vi "extract_exe.vi"(4 "files_to_extract (relative) []":path[](array[path]), 6 "quiet?":bool=TRUE, 8 "error in (no error)":errorcluster, 9 "preview?":bool, 10 "target_path in":path, 11 "archive_path (file_dialog)":path) -> (0 "error out":errorcluster, 1 "files []":path[](array[path]), 2 "target_path out":path, 3 "archive_path out":path)   [LabVIEW 2015, in "lv-bin-7zip.lvlib"]
uses:
  lv-bin-7zip.lvlib
  <userlib>/antonio-alexander/lv-bin/public/api/v1/v1.lvlib
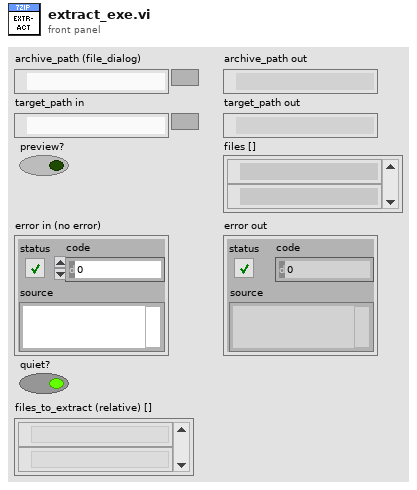
[diagram p1: front panel]
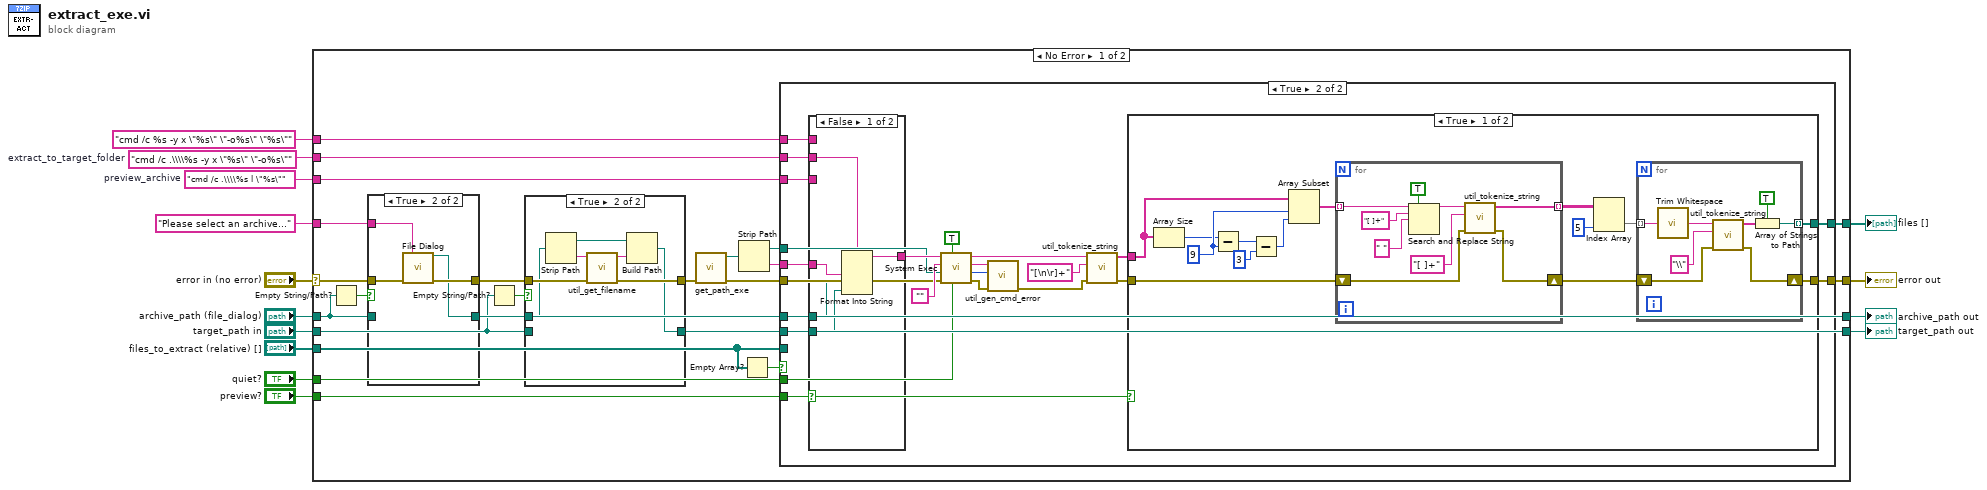
[diagram p0: block diagram]
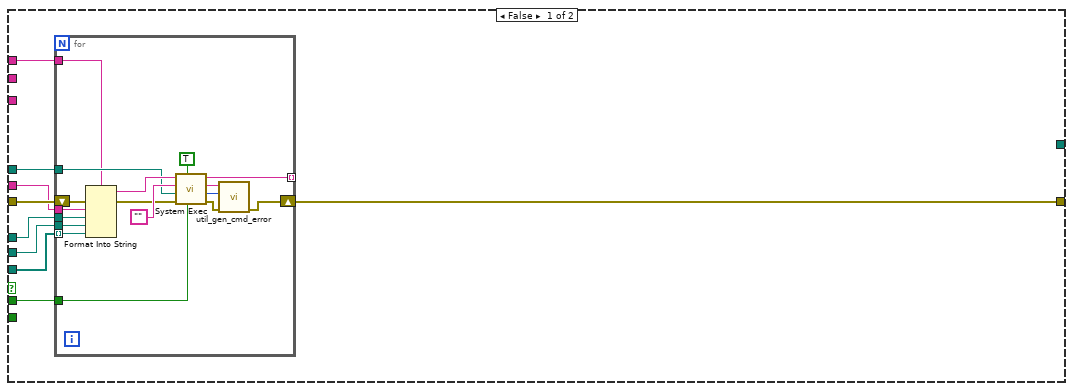
[diagram p4: hidden frame]
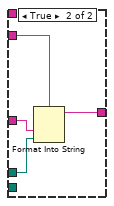
[diagram p5: hidden frame]
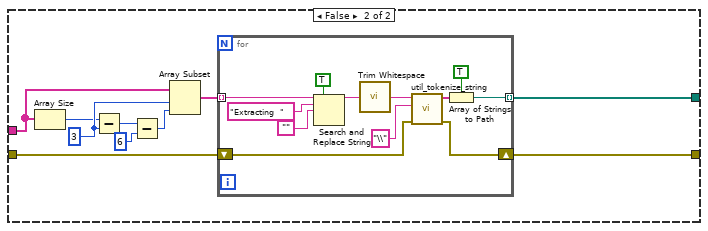
[diagram p6: hidden frame]
diagram:
  w5 = "cmd /c .\\\\%s l \"%s\""  # preview_archive
  w6 = "cmd /c .\\\\%s -y x \"%s\" \"-o%s\""  # extract_to_target_folder
  n1 = case shown="No Error" "error in (no error)" {
    selector: "error in (no error)" -> [w34 w163]
    tunnel: [w22 w163] -> w13
    tunnel: "target_path in" -> [w20 _]
    tunnel: "archive_path (file_dialog)" -> [w33 _]
    tunnel: "Please select an archive..." ("prompt") -> [w31 _]
    tunnel: [w23 _] -> w9
    tunnel: [w21 _] -> w8
    tunnel: "preview?" -> [w25 _]
    tunnel: w6 -> [w27 _]
    tunnel: w5 -> [w26 _]
    tunnel: [w24 _] -> w4
    tunnel: "quiet?" -> [w19 _]
    tunnel: "cmd /c %s -y x \"%s\" \"-o%s\" \"%s\"" ("format string") -> [w18 _]
    tunnel: "files_to_extract (relative) []" -> [w17 _]
    frame No Error {
      n2 = Empty String/Path?(string/path=w33) -> (empty?=w32:bool)
      n3 = case shown="True" w32 {
        tunnel: w34 -> [w47 w52]
        tunnel: [w47 w51] -> w29
        tunnel: w33 -> [w48 _]
        tunnel: w31 -> [_ w50]
        tunnel: [w48 w49] -> w21
        frame False {
        }
        frame True {
          n4 = call "File Dialog"("prompt"=w50, "error in"=w52) -> ("selected path"=w49:path, "error out"=w51:errorcluster)  [unwired: 10 in, 2 out]
        }
      }
      n5 = Empty String/Path?(string/path=w20) -> (empty?=w30:bool)
      n6 = case shown="True" w30 {
        tunnel: w29 -> [w38 w45]
        tunnel: w21 -> [_ w41]
        tunnel: w20 -> [w39 _]
        tunnel: [w39 w40] -> w23
        tunnel: [w38 w42] -> w28
        frame False {
        }
        frame True {
          n7 = Strip Path(path=w41) -> (stripped path=w44:path, name=w46:string)
          n8 = call "util_get_filename.vi"("error in (no error)"=w45, "filename_with_extension"=w46) -> ("error out"=w42:errorcluster, "filename_without_extension"=w43:string)  [unwired: 8 in]
          n9 = Build Path(base path=w44, name or relative path=w43) -> (appended path=w40:path)
        }
      }
      n10 = call "get_path_exe.vi"("error in (no error)"=w28) -> ("error out"=w15:errorcluster, "exe"=w37:path)  [unwired: 9 in]
      n11 = Strip Path(path=w37) -> (stripped path=w35:path, name=w36:string)
      n12 = Empty Array?(array=w17) -> (empty?=w16:bool)
      n13 = case shown="True" w16 {
        tunnel: w36 -> [w58 w97]
        tunnel: w35 -> [w54 w96]
        tunnel: w27 -> [_ w94]
        tunnel: w26 -> [_ w93]
        tunnel: w25 -> [_ w92]
        tunnel: [_ w91] -> w24
        tunnel: w23 -> [w56 w90]
        tunnel: [w59 w89] -> w22
        tunnel: w21 -> [w57 w82]
        tunnel: w15 -> [w61 w81]
        tunnel: w19 -> [w53 w79]
        tunnel: w18 -> [w60 w78]
        tunnel: w17 -> [w55 _]
        frame False {
          n14 = for {
            tunnel: w54 -> [w73]
            tunnel: w56 -> [w72]
            tunnel: w57 -> [w71]
            tunnel: w58 -> [w74]
            tunnel: [w66] -> _ mode=indexing
            tunnel: w55 -> [w68] mode=indexing
            tunnel: w60 -> [w67]
            shift-right: [w69] -> w59
            shift-left: w61 -> [w62]
            tunnel: w53 -> [w63]
            n15 = Format Into String(format string=w67, w74, w71, w72, w68) -> (resulting string=w77:string)  [unwired: 2 in, 1 out]
            n16 = call <vilib>:"System Exec.vi"("run minimized? (F)"=w63, "wait until completion? (T)"=TRUE, "error in (no error)"=w62, "working directory"=w73, "standard input"="", "command line"=w77) -> ("error out"=w70:errorcluster, "return code"=w64:i32, "standard error"=w65:string, "standard output"=w66:string)  [unwired: 2 in]
            n17 = call <userlib>:"util_gen_cmd_error.vi"("error in (no error)"=w70, "return_code"=w64, "standard_error"=w65) -> ("error out"=w69:errorcluster)  [unwired: 8 in]
          }
        }
        frame True {
          n18 = case shown="False" w92 {
            tunnel: [w105 w109] -> w100
            tunnel: w97 -> [w104 w108]
            tunnel: w90 -> [w103 _]
            tunnel: w82 -> [w102 w107]
            tunnel: w94 -> [w101 _]
            tunnel: w93 -> [_ w106]
            tunnel: w78 -> [_ _]
            frame False {
              n19 = Format Into String(format string=w101, w104, w102, w103) -> (resulting string=w105:string)  [unwired: 2 in, 1 out]
            }
            frame True {
              n20 = Format Into String(format string=w106, w108, w107) -> (resulting string=w109:string)  [unwired: 2 in, 1 out]
            }
          }
          n21 = call <vilib>:"System Exec.vi"("run minimized? (F)"=w79, "wait until completion? (T)"=TRUE, "error in (no error)"=w81, "working directory"=w96, "standard input"="", "command line"=w100) -> ("error out"=w95:errorcluster, "return code"=w80:i32, "standard error"=w83:string, "standard output"=w87:string)  [unwired: 2 in]
          n22 = call <userlib>:"util_gen_cmd_error.vi"("error in (no error)"=w95, "return_code"=w80, "standard_error"=w83) -> ("error out"=w86:errorcluster)  [unwired: 8 in]
          n23 = call <userlib>:"util_tokenize_string.vi"("error in (no error)"=w86, "delimiter"="[\n\r]+" ("delimiter ([\\s\\t\\n\\r]+)"), "input_string"=w87) -> ("error out"=w85:errorcluster, "before_match []"=w84:string[])  [unwired: 6 in, 1 out]
          n24 = case shown="True" w92 {
            tunnel: [w114 w143] -> w91
            tunnel: w85 -> [w110 w141]
            tunnel: [w112 w144] -> w89
            tunnel: w84 -> [w111 w142]
            frame True {
              w119 = 9 ("length")
              n25 = Array Size(array=w111) -> (size(s)=w118:i32)
              n26 = Subtract(x=w118, y=w119) -> (x-y=w120:i32)
              n27 = Subtract(x=w120, y=3 ("x")) -> (x-y=w121:i32)
              n28 = Array Subset(array=w111, index=w119, length=w121) -> (w123:string[])
              n29 = for {
                tunnel: w123 -> [w132] mode=indexing
                tunnel: [w126] -> w117 mode=indexing
                shift-right: [w124] -> w113
                shift-left: w110 -> [w125]
                n30 = Search and Replace String(replace all?=TRUE ("replace all? (F)"), input string=w132, search string="[ ]+", replace string=" " ("replace string (\"\")")) -> (result string=w127:string)  [unwired: 4 in, 3 out]
                n31 = call <userlib>:"util_tokenize_string.vi"("error in (no error)"=w125, "delimiter"="[ ]+" ("delimiter ([\\s\\t\\n\\r]+)"), "input_string"=w127) -> ("error out"=w124:errorcluster, "before_match []"=w126:string[])  [unwired: 6 in, 1 out]
              }
              n32 = Index Array(array=w117, index (col)=5 ("disabled index (col)")) -> (element=w115:string[])  [unwired: 1 in]
              n33 = for {
                tunnel: w115 -> [w140] mode=indexing
                tunnel: [w137] -> w114 mode=indexing
                shift-right: [w133] -> w112
                shift-left: w113 -> [w134]
                n34 = call <vilib>:"Trim Whitespace.vi"("string"=w140) -> ("trimmed string"=w139:string)  [unwired: 1 in]
                n35 = call <userlib>:"util_tokenize_string.vi"("error in (no error)"=w134, "delimiter"="\\" ("delimiter ([\\s\\t\\n\\r]+)"), "input_string"=w139) -> ("error out"=w133:errorcluster, "before_match []"=w138:string[])  [unwired: 6 in, 1 out]
                n36 = Array of Strings to Path(0:w138, 1:TRUE ("relative")) -> (2:w137:path)
              }
            }
            frame False {
              w146 = 3 ("length")
              n37 = Array Size(array=w142) -> (size(s)=w145:i32)
              n38 = Subtract(x=w145, y=w146) -> (x-y=w147:i32)
              n39 = Subtract(x=w147, y=6 ("x")) -> (x-y=w148:i32)
              n40 = Array Subset(array=w142, index=w146, length=w148) -> (w150:string[])
              n41 = for {
                tunnel: w150 -> [w162] mode=indexing
                tunnel: [w153] -> w143 mode=indexing
                shift-right: [w151] -> w144
                shift-left: w141 -> [w152]
                n42 = Search and Replace String(replace all?=TRUE ("replace all? (F)"), input string=w162, search string="Extracting  ", replace string="") -> (result string=w154:string)  [unwired: 4 in, 3 out]
                n43 = call <vilib>:"Trim Whitespace.vi"("string"=w154) -> ("trimmed string"=w155:string)  [unwired: 1 in]
                n44 = call <userlib>:"util_tokenize_string.vi"("error in (no error)"=w152, "delimiter"="\\" ("delimiter ([\\s\\t\\n\\r]+)"), "input_string"=w155) -> ("error out"=w151:errorcluster, "before_match []"=w156:string[])  [unwired: 6 in, 1 out]
                n45 = Array of Strings to Path(0:w156, 1:TRUE ("relative")) -> (2:w153:path)
              }
            }
          }
        }
      }
    }
    frame Error {
    }
  }
  "error out" <- w13
  "archive_path out" <- w8
  "target_path out" <- w9
  "files []" <- w4
